vi "HDI Bond Pad BL Match.vi"(9 "error in (no error)":errorcluster, 10 "Image Src":T1) -> (0 "error out":errorcluster, 1 "In Range?":bool, 2 "y rel move":dbl, 3 "x rel move":dbl, 5 "Angle Between Lines":dbl)   [LabVIEW 2011]
uses:
  <vilib>/vision/Image Controls.llb/IMAQ Image.ctl
  <vilib>/vision/NI_Vision_Development_Module.lvlib
panel:
  in  "Scale Factor":sgl=0.000429
  out "y":sgl
  out "x":sgl
  out "X Coordinate Pixels":dbl
  out "Y Coordinate Pixels":sgl
  out "Remaining Outputs":T2 {"Horizontal calibrated"."Point2"."Y" format="%.2f"; "Horizontal calibrated"."Point2"."X" format="%.2f"; "Horizontal calibrated"."Point1"."Y" format="%.2f"; "Horizontal calibrated"."Point1"."X" format="%.2f"; "Horizontal"."Point2"."Y" format="%.2f"; "Horizontal"."Point2"."X" format="%.2f"; "Horizontal"."Point1"."Y" format="%.2f"; "Horizontal"."Point1"."X" format="%.2f"; "Edge Coordinates (calibrated) (Straight Edge (Rake) 2)"."Y" format="%.2f"; "Edge Coordinates (calibrated) (Straight Edge (Rake) 2)"."X" format="%.2f"; "Edge Coordinates (Straight Edge (Rake) 2)"."Y" format="%.2f"; "Edge Coordinates (Straight Edge (Rake) 2)"."X" format="%.2f"}
  out "Image Out":T1(plugin-control)
  out "Vertical Calibrated":T3 {"Point2"."Y" format="%.2f"; "Point2"."X" format="%.2f"; "Point1"."Y" format="%.2f"; "Point1"."X" format="%.2f"}
  out "Hori":cluster{"X":sgl, "Y":sgl}[](array[cluster]) {"Y" format="%.2f"; "X" format="%.2f"}
  out "Vertical rake":T3 {"Point2"."Y" format="%.2f"; "Point2"."X" format="%.2f"; "Point1"."Y" format="%.2f"; "Point1"."X" format="%.2f"}
  out "Edge Coordinates (Straight Edge (Rake) 1)":cluster{"X":sgl, "Y":sgl}[](array[cluster]) {"Y" format="%.2f"; "X" format="%.2f"}
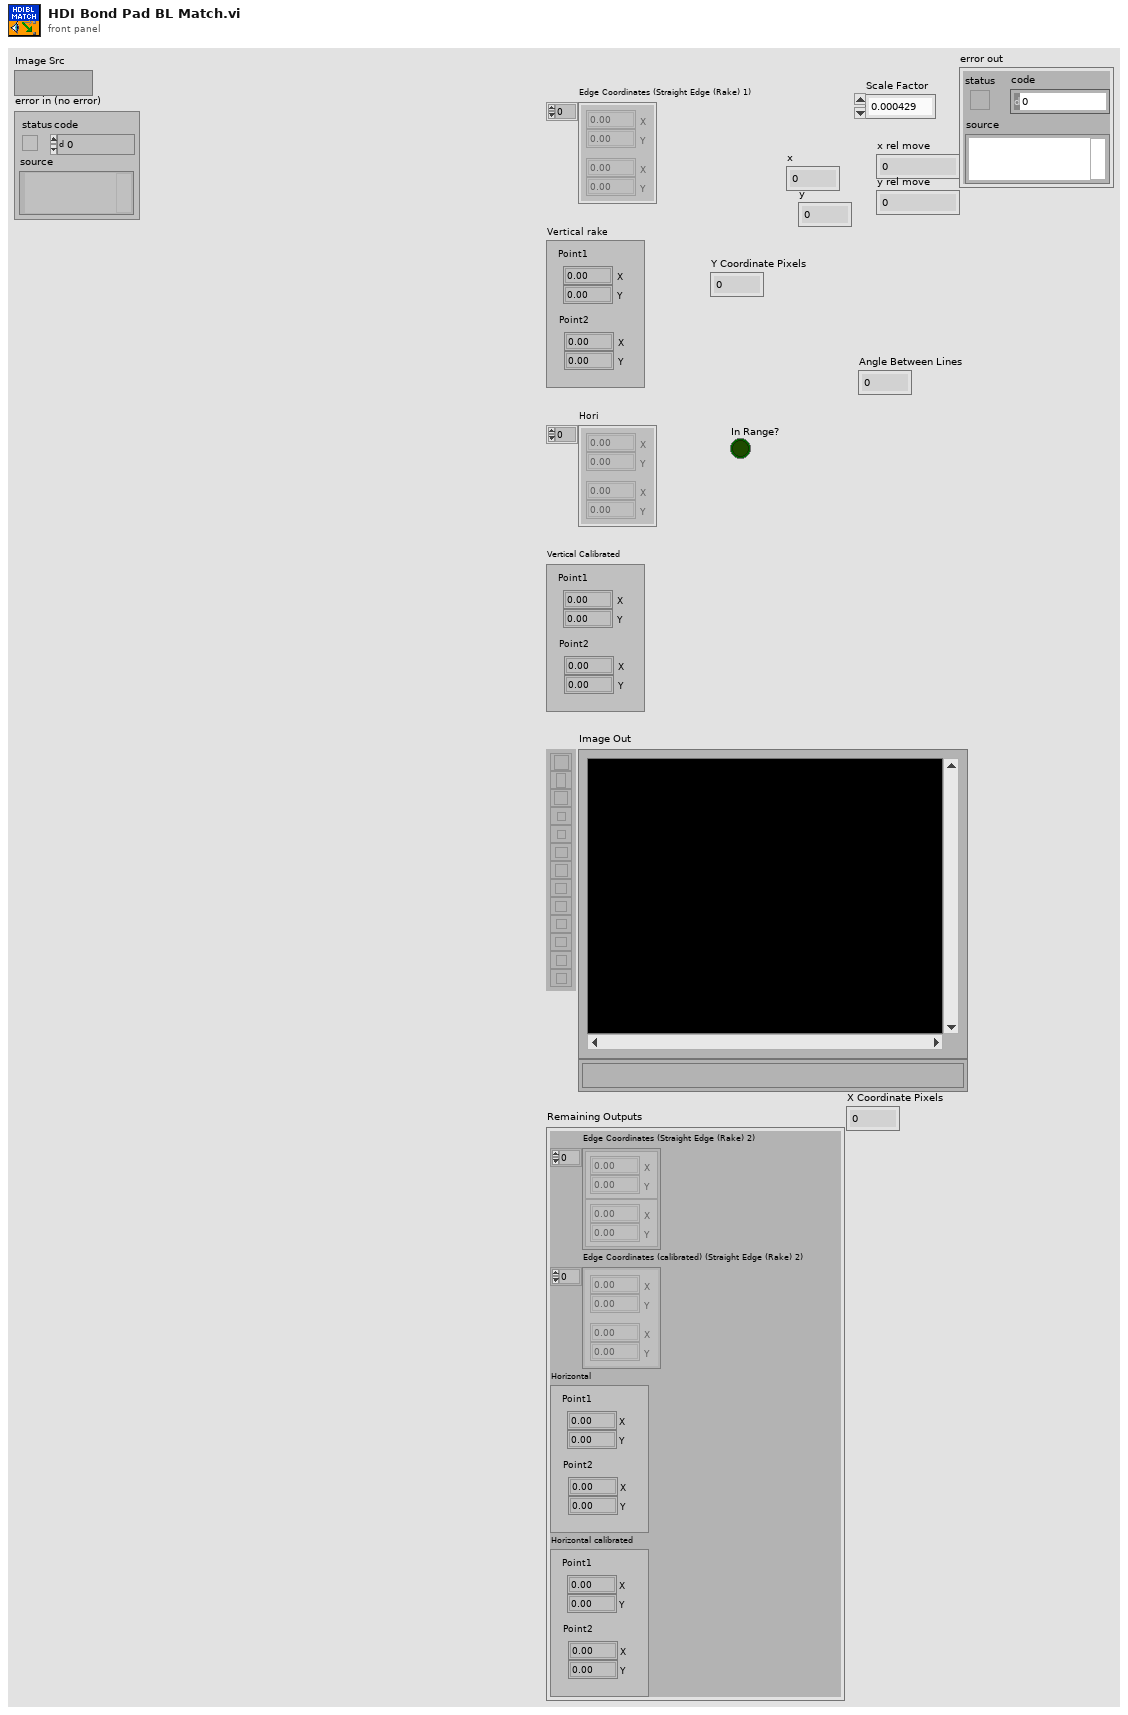
[diagram p1: front panel]
types:
  T1 = typedef "IMAQ Image.ctl" = refnum<image>
  T2 = cluster{"Edge Coordinates (Straight Edge (Rake) 2)":cluster{"X":sgl, "Y":sgl}[], "Edge Coordinates (calibrated) (Straight Edge (Rake) 2)":cluster{"X":sgl, "Y":sgl}[], "Horizontal":cluster{"Point1":cluster{"X":sgl, "Y":sgl}, "Point2":cluster{"X":sgl, "Y":sgl}}, "Horizontal calibrated":cluster{"Point1":cluster{"X":sgl, "Y":sgl}, "Point2":cluster{"X":sgl, "Y":sgl}}}
  T3 = cluster{"Point1":cluster{"X":sgl, "Y":sgl}, "Point2":cluster{"X":sgl, "Y":sgl}}
  T4 = cluster{"Global Rectangle":i32[], "Contours":cluster{"ID":enum32{"External", "Internal"}, "Type":u32, "Coordinates":i32[]}[]}
  T5 = cluster{"Contrast":i32, "Filter width":i32, "Steepness":i32, "Subsampling Ratio":u32, "Scan Direction":u32, "Show Search Area":bool, "Show Search Lines":bool, "Show Edges Found":bool, "Show Result":bool}
  T6 = typedef "IMAQ Rectangle" = cluster{"Left":i32, "Top":i32, "Right":i32, "Bottom":i32, "Rotation":dbl}
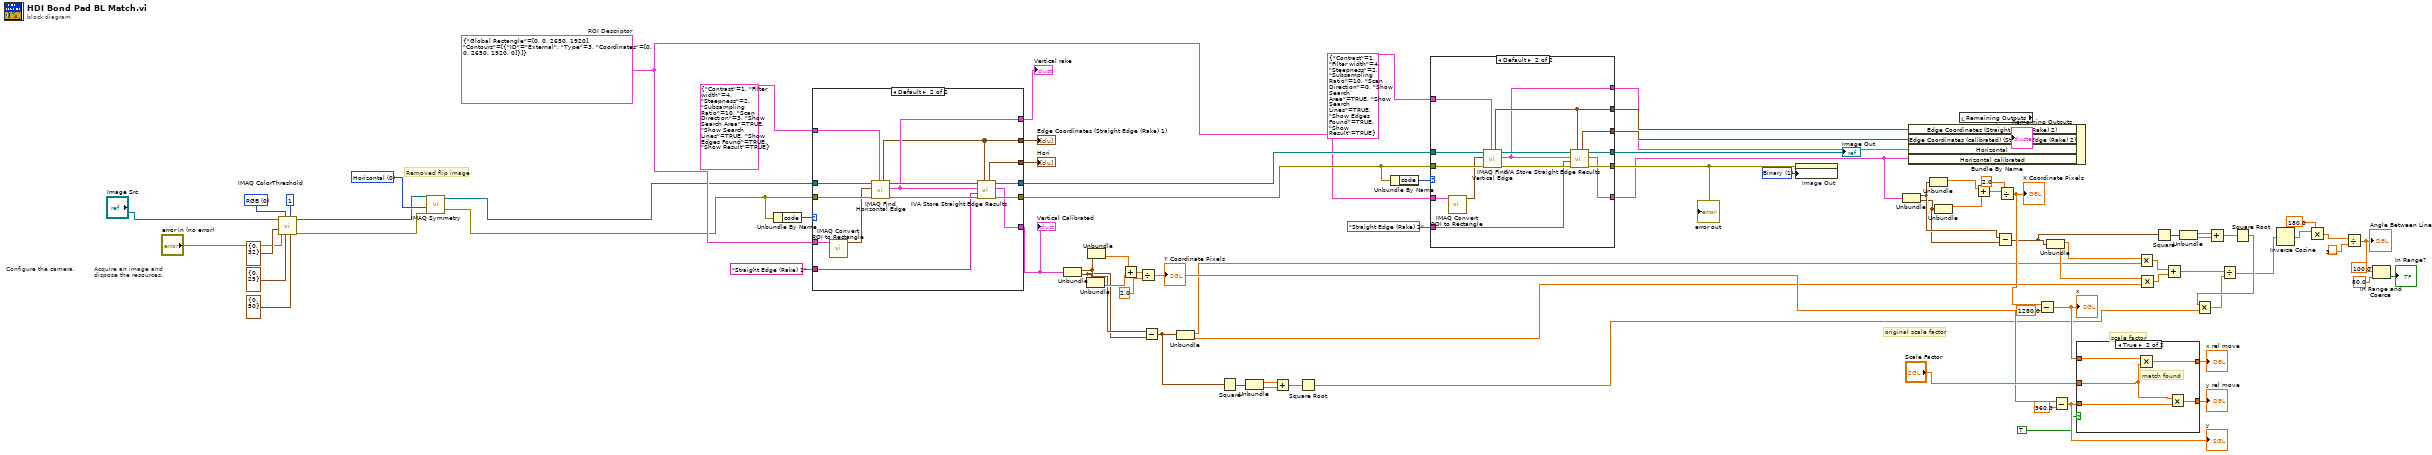
[diagram p0: block diagram]
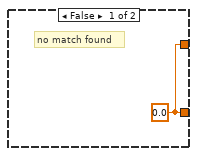
[diagram p2: hidden frame]
diagram:
  w5 = u32 0 items=["Horizontal", "Vertical", "Central", "1st Diagonal", "2nd Diagonal"] ("Type of Symmetry")
  w6 = T4 {"Global Rectangle"=[0, 0, 2650, 1920], "Contours"=[{"ID"=enum."External", "Type"=3, "Coordinates"=[0, 0, 2650, 1920, 0]}]}  # ROI Descriptor
  w64 = u32 1 items=["Grayscale", "Binary", "Gradient", "Rainbow", "Temperature", "User Defined"] ("Palette")
  w84 = u16 0 items=["RGB", "HSL", "HSV", "HSI"] ("Color Mode")
  # "Removed flip image"
  # "original scale factor"
  # "scale factor"
  # "Acquire an image and\ndispose the resources."
  # "Configure the camera."
  n1 = call "IMAQ ColorThreshold"("Blue or Luma or Val or Inten Range"=cluster{"Lower value":i32, "Upper value":i32} {"Lower value"=0, "Upper value"=50}, "Replace Value"=1, "Green or Sat Range"=cluster{"Lower value":i32, "Upper value":i32} {"Lower value"=0, "Upper value"=25}, "Color Mode"=w84, "error in (no error)"="error in (no error)", "Red or Hue Range"=cluster{"Lower value":i32, "Upper value":i32} {"Lower value"=0, "Upper value"=32}, "Image Src"="Image Src") -> ("error out"=w2:errorcluster, "Image Dst Out"=w4:T1)  [unwired: 3 in]
  n2 = call "IMAQ Symmetry"("error in (no error)"=w2, "Type of Symmetry"=w5, "Image Src"=w4) -> ("error out"=w1:errorcluster, "Image Dst Out"=w3:T1)  [unwired: 2 in]
  n3 = Unbundle By Name(w1) -> ("code"=w74:i32)
  n4 = case shown="Default" w74 {
    tunnel: T5 {"Contrast"=1, "Filter width"=4, "Steepness"=2, "Subsampling Ratio"=10, "Scan Direction"=3, "Show Search Area"=TRUE, "Show Search Lines"=TRUE, "Show Edges Found"=TRUE, "Show Result"=TRUE} ("Settings (Straight Edge (Rake) 1)") -> [_ w100]
    tunnel: w3 -> [w86 w99]
    tunnel: w1 -> [_ w98]
    tunnel: w6 -> [_ w97]
    tunnel: [w86 w94] -> w73
    tunnel: [_ w92] -> w79
    tunnel: [_ w91] -> w78
    tunnel: [_ w90] -> w77
    tunnel: "Straight Edge (Rake) 1" ("Step Name") -> [_ w89]
    tunnel: [_ w88] -> w75
    tunnel: [_ w87] -> w61
    frame -1074396199, -1074396198 {
      # "Discard Coordinate System Error"
    }
    frame Default {
      n5 = call "IMAQ Convert ROI to Rectangle"("ROI Descriptor"=w97) -> ("Rectangle"=w96:T6)  [unwired: 8 in, 1 out]
      n6 = call "IMAQ Find Horizontal Edge"("Settings"=w100, "error in (no error)"=w98, "Rectangle"=w96, "Image"=w99) -> ("error out"=w93:errorcluster, "Line Coordinates"=w91:T3, "Image Out"=w95:T1, "Edge Coordinates"=w90:cluster{"X":sgl, "Y":sgl}[])  [unwired: 2 in, 2 out]
      n7 = call <vilib>:"IVA Store Straight Edge Results.vi"("Edge Coordinates"=w90, "error in (no error)"=w93, "Step Name"=w89, "Line Coordinates"=w91, "Image in"=w95) -> ("error out"=w92:errorcluster, "Line Coordinates (calibrated)"=w87:T3, "Image dup"=w94:T1, "Edge Coordinates (calibrated)"=w88:cluster{"X":sgl, "Y":sgl}[])  [unwired: 3 in]
    }
  }
  "Edge Coordinates (Straight Edge (Rake) 1)" <- w77
  "Vertical rake" <- w78
  "Hori" <- w75
  "Vertical Calibrated" <- w61
  n8 = Unbundle(w61) -> ("Point1"=w39:cluster{"X":sgl, "Y":sgl}, "Point2"=w38:cluster{"X":sgl, "Y":sgl})
  n9 = Unbundle(w38) -> ("Y"=w59:sgl)  [unwired: 1 out]
  n10 = Unbundle(w39) -> ("Y"=w60:sgl)  [unwired: 1 out]
  n11 = Add(x=w60, y=w59) -> (x+y=w58:sgl)
  n12 = Divide(x=w58, y=sgl 2.0) -> (x/y=w44:sgl)
  "Y Coordinate Pixels" <- w44
  n13 = Subtract(x=w39, y=w38) -> (x-y=w22:cluster{"X":sgl, "Y":sgl})
  n14 = Unbundle(w22) -> ("X"=w35:sgl, "Y"=w34:sgl)
  n15 = Square(x=w22) -> (x^2=w26:cluster{"X":sgl, "Y":sgl})
  n16 = Unbundle(w26) -> ("X"=w25:sgl, "Y"=w24:sgl)
  n17 = Add(x=w25, y=w24) -> (x+y=w23:sgl)
  n18 = Square Root(x=w23) -> (sqrt(x)=w19:sgl)
  n19 = Unbundle By Name(w79) -> ("code"=w66:i32)
  n20 = case shown="Default" w66 {
    tunnel: w73 -> [w101 w115]
    tunnel: w79 -> [_ w114]
    tunnel: T5 {"Contrast"=1, "Filter width"=4, "Steepness"=2, "Subsampling Ratio"=10, "Scan Direction"=0, "Show Search Area"=TRUE, "Show Search Lines"=TRUE, "Show Edges Found"=TRUE, "Show Result"=TRUE} ("Settings (Straight Edge (Rake) 2)") -> [_ w113]
    tunnel: w6 -> [_ w112]
    tunnel: [w101 w109] -> w65
    tunnel: [_ w107] -> w71
    tunnel: [_ w106] -> w70
    tunnel: [_ w105] -> w69
    tunnel: [_ w104] -> w56
    tunnel: [_ w103] -> w68
    tunnel: "Straight Edge (Rake) 2" ("Step Name") -> [_ w102]
    frame -1074396199, -1074396198 {
      # "Discard Coordinate System Error"
    }
    frame Default {
      n21 = call "IMAQ Convert ROI to Rectangle"("ROI Descriptor"=w112) -> ("Rectangle"=w111:T6)  [unwired: 8 in, 1 out]
      n22 = call "IMAQ Find Vertical Edge"("Settings"=w113, "error in (no error)"=w114, "Rectangle"=w111, "Image"=w115) -> ("error out"=w108:errorcluster, "Line Coordinates"=w103:T3, "Image Out"=w110:T1, "Edge Coordinates"=w106:cluster{"X":sgl, "Y":sgl}[])  [unwired: 2 in, 2 out]
      n23 = call <vilib>:"IVA Store Straight Edge Results.vi"("Edge Coordinates"=w106, "error in (no error)"=w108, "Step Name"=w102, "Line Coordinates"=w103, "Image in"=w110) -> ("error out"=w107:errorcluster, "Line Coordinates (calibrated)"=w104:T3, "Image dup"=w109:T1, "Edge Coordinates (calibrated)"=w105:cluster{"X":sgl, "Y":sgl}[])  [unwired: 3 in]
    }
  }
  "Image Out" <- w65
  "error out" <- w71
  n24 = property on="Image Out" class="ImageControl"(error in=w71, "Palette:Palette Type"=w64) -> ()  [unwired: 1 in, 2 out]
  n25 = Unbundle(w56) -> ("Point1"=w41:cluster{"X":sgl, "Y":sgl}, "Point2"=w40:cluster{"X":sgl, "Y":sgl})
  n26 = Unbundle(w41) -> ("X"=w53:sgl)  [unwired: 1 out]
  n27 = Unbundle(w40) -> ("X"=w52:sgl)  [unwired: 1 out]
  n28 = local read "Remaining Outputs"() -> (w62:T2)
  n29 = Bundle By Name(cluster=w62, "Edge Coordinates (Straight Edge (Rake) 2)"=w70, "Edge Coordinates (calibrated) (Straight Edge (Rake) 2)"=w69, "Horizontal"=w68, "Horizontal calibrated"=w56) -> (→"Remaining Outputs":T2)
  n30 = Add(x=w53, y=w52) -> (x+y=w55:sgl)
  n31 = Subtract(x=w41, y=w40) -> (x-y=w31:cluster{"X":sgl, "Y":sgl})
  n32 = Divide(x=w55, y=2.0) -> (x/y=w43:dbl)
  "X Coordinate Pixels" <- w43
  n33 = Subtract(x=w43, y=sgl 1280.0) -> (x-y=w48:dbl)
  "x" <- w48
  n34 = Unbundle(w31) -> ("X"=w37:sgl, "Y"=w36:sgl)
  n35 = Subtract(x=w44, y=sgl 960.0) -> (x-y=w49:sgl)
  "y" <- w49
  n36 = case shown="True" TRUE {
    tunnel: w49 -> [_ w121]
    tunnel: w48 -> [_ w120]
    tunnel: [w116 w119] -> w47
    tunnel: [w116 w118] -> w46
    tunnel: "Scale Factor" -> [_ w117]
    frame False {
      w116 = sgl 0.0
      # "no match found"
    }
    frame True {
      # "match found"
      n37 = Multiply(x=w120, y=w117) -> (x*y=w119:dbl)
      n38 = Multiply(x=w117, y=w121) -> (x*y=w118:sgl)
    }
  }
  "x rel move" <- w47
  "y rel move" <- w46
  n39 = Multiply(x=w37, y=w35) -> (x*y=w33:sgl)
  n40 = Multiply(x=w36, y=w34) -> (x*y=w32:sgl)
  n41 = Square(x=w31) -> (x^2=w30:cluster{"X":sgl, "Y":sgl})
  n42 = Add(x=w33, y=w32) -> (x+y=w21:sgl)
  n43 = Unbundle(w30) -> ("X"=w29:sgl, "Y"=w28:sgl)
  n44 = Add(x=w29, y=w28) -> (x+y=w27:sgl)
  n45 = Square Root(x=w27) -> (sqrt(x)=w20:sgl)
  n46 = Multiply(x=w20, y=w19) -> (x*y=w18:sgl)
  n47 = Divide(x=w21, y=w18) -> (x/y=w17:sgl)
  n48 = Inverse Cosine(1:w17) -> (0:w16:sgl)
  n49 = Multiply(x=w16, y=sgl 180.0) -> (x*y=w14:sgl)
  n50 = Divide(x=w14, y=3.141592653589793) -> (x/y=w12:dbl)
  "Angle Between Lines" <- w12
  n51 = In Range and Coerce(upper limit=100.0, x=w12, lower limit=80.0) -> (In Range?=→"In Range?":bool)  [unwired: 1 out]
